vi "CompressorSpeed.vi"(6 "Max Speed":dbl, 7 "Min Speed":dbl, 9 "Reinitialize Controller":bool, 10 "Controller Toggle P 2":bool, 11 "Compressor Input":T2={"Compressor Speed Adjust"=100.0, "Accept Autotune Water Pump"=FALSE, "Fine slide in P"=refnum, "file for water pump"=path "", "autotune? water pump"=FALSE, "PID gains in water pump"={"proportional gain (Kc)"=0.0, "integral time (Ti, min)"=0.0, "derivative time (Td, min)"=0.0}} {"Compressor Speed Adjust" min=0.0 max=240.0 step=1.0 scale=0.0..240.0}) -> (2 "output to valve":dbl, 3 "output cluster":T1)   [LabVIEW 2017]
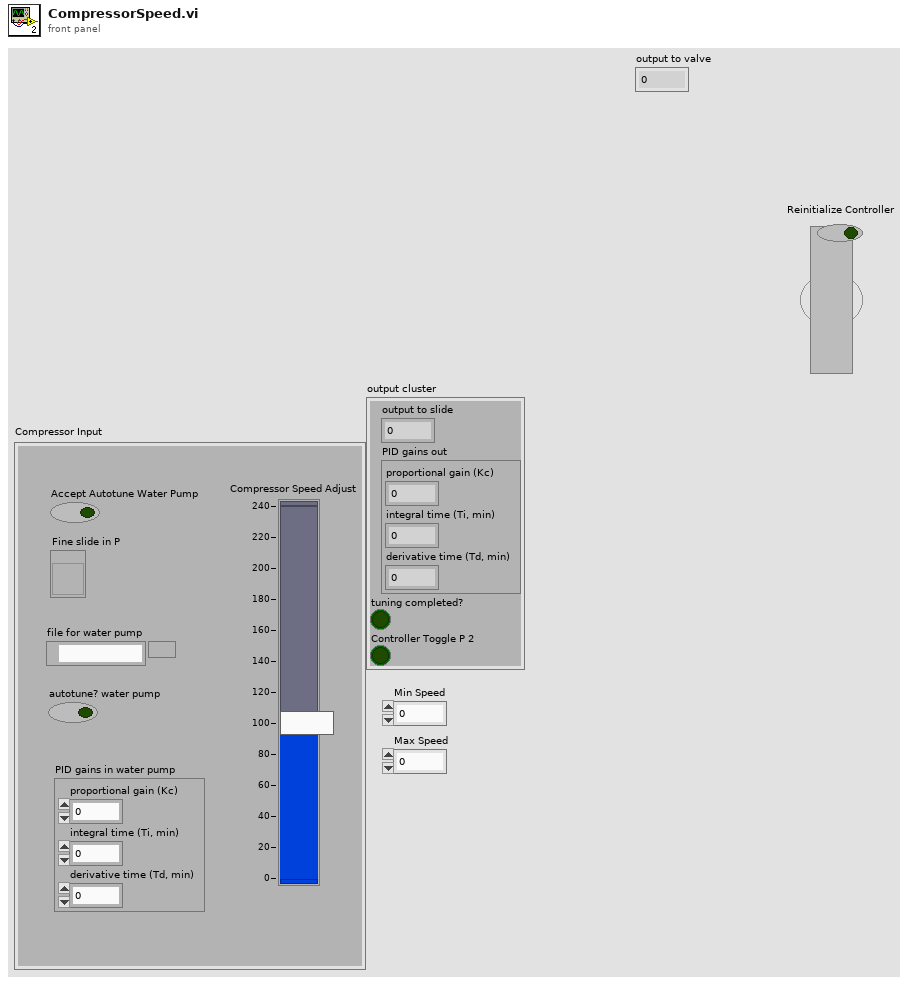
[diagram p1: front panel]
types:
  T1 = cluster{"output to slide":dbl, "PID gains out":cluster{"proportional gain (Kc)":dbl, "integral time (Ti, min)":dbl, "derivative time (Td, min)":dbl}, "tuning completed?":bool, "Controller Toggle P 2":bool}
  T2 = cluster{"Compressor Speed Adjust":dbl, "Accept Autotune Water Pump":bool, "Fine slide in P":refnum<vi>, "file for water pump":path, "autotune? water pump":bool, "PID gains in water pump":cluster{"proportional gain (Kc)":dbl, "integral time (Ti, min)":dbl, "derivative time (Td, min)":dbl}}
  T3 = cluster{"proportional gain (Kc)":dbl, "integral time (Ti, min)":dbl, "derivative time (Td, min)":dbl}
  T4 = enum8{"Enabled", "Disabled", "Disabled and Grayed Out"}
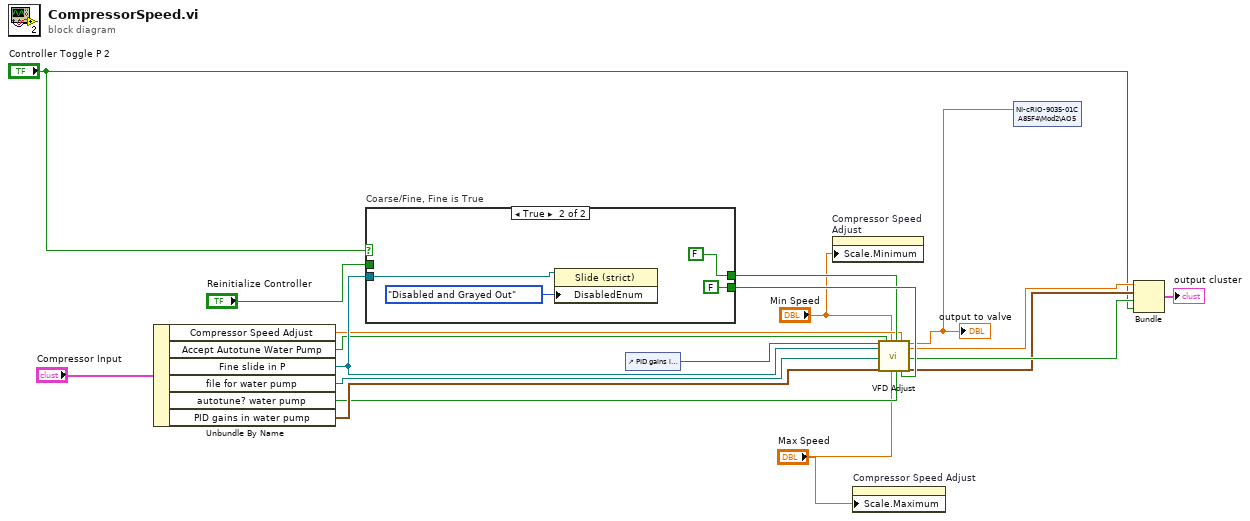
[diagram p0: block diagram]
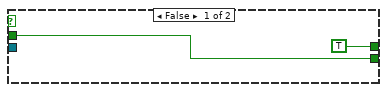
[diagram p2: hidden frame]
diagram:
  n1 = Unbundle By Name("Compressor Input") -> ("Compressor Speed Adjust"=w9:dbl, "Accept Autotune Water Pump"=w11:bool, "Fine slide in P"=w15:refnum<vi>, "file for water pump"=w16:path, "autotune? water pump"=w12:bool, "PID gains in water pump"=w17:T3)
  n2 = case "Coarse/Fine, Fine is True" shown="True" "Controller Toggle P 2" {
    tunnel: "Reinitialize Controller" -> [w20 _]
    tunnel: [w20 FALSE] -> w13
    tunnel: [TRUE FALSE] -> w10
    tunnel: w15 -> [_ w23]
    frame False {
    }
    frame True {
      n3 = property on="Property Node" class="Slide (strict)"(reference=w23, "DisabledEnum"=T4."Disabled and Grayed Out" ("Disabled")) -> ()  [unwired: 1 in, 2 out]
    }
  }
  n4 = control-ref of="PID gains in water pump"() -> (w14:refnum<vi>)
  n5 = property on="Compressor Speed Adjust" class="Slide (strict)"("Scale.Minimum"="Min Speed") -> ()  [unwired: 2 in, 2 out]
  n6 = property on="Compressor Speed Adjust" class="Slide (strict)"("Scale.Maximum"="Max Speed") -> ()  [unwired: 2 in, 2 out]
  n7 = call "VFD Adjust.vi"("PID Gains Cluster Ref"=w14, "Slide Refnum in"=w15, "file (use dialog)"=w16, "PID gains"=w17, "Accept Autotune"=w11, "Min Speed"="Min Speed", "Max Speed"="Max Speed", "Controller Toggle (Manual Mode)"=w10, "autotune? (F)"=w12, "Valve Manual Adjust"=w9, "Reinitialize Controller"=w13) -> ("output to valve"=w3:dbl, "output to slide"=w8:dbl, "tuning completed?"=w7:bool, "PID gains out"=w6:T3)  [unwired: 4 in, 1 out]
  "output to valve" <- w3
  n8 = shared-variable "NI-cRIO-9035-01CA85F4\\Mod2\\AO5"(w3) -> ()  [unwired: 1 in, 1 out]
  n9 = Bundle("output to slide"=w8, "PID gains out"=w6, "tuning completed?"=w7, "Controller Toggle P 2"="Controller Toggle P 2") -> (→"output cluster":T1)  [unwired: 1 in]
